vi "FlatToRichcif_manager_PluginConfig.vi"(5 "OutputClusterType":T1, 11 "InputCluster":T2) -> (3 "OutputCluster":T1)   [LabVIEW 2021, in "CIF_Launcher_client.lvlib"]
uses:
  CIF_Launcher_client.lvlib
  cif_manager_PluginConfig_Flat.ctl
  cif_manager_PluginConfig.ctl
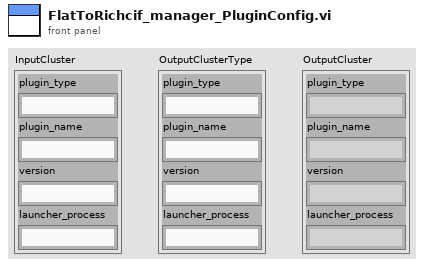
[diagram p1: front panel]
types:
  T1 = typedef "CIF_Launcher_client.lvlib/cif_manager_PluginConfig.ctl" = cluster{"plugin_type":string, "plugin_name":string, "version":string, "launcher_process":string}
  T2 = typedef "CIF_Launcher_client.lvlib/cif_manager_PluginConfig_Flat.ctl" = cluster{"plugin_type":string, "plugin_name":string, "version":string, "launcher_process":string}
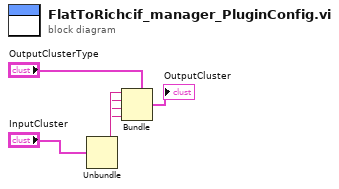
[diagram p0: block diagram]
diagram:
  n1 = Unbundle "Unbundle"("InputCluster") -> ("plugin_type"=w4:string, "plugin_name"=w3:string, "version"=w2:string, "launcher_process"=w1:string)
  n2 = Bundle "Bundle"(cluster="OutputClusterType", "plugin_type"=w4, "plugin_name"=w3, "version"=w2, "launcher_process"=w1) -> (→"OutputCluster":T1)
